vi "C867_Macro_Test.vi"() -> ()   [LabVIEW 2026]
panel:
  out "BOOL 5":i32
  out "BOOL 4":i32
  out "BOOL 3":i32
  out "BOOL 2":i32
  out "BOOL":i32
  out "szAnswer":string
  out "error out":errorcluster caption="sortie d'erreur"
  in  "error in":errorcluster caption="entrée d'erreur"
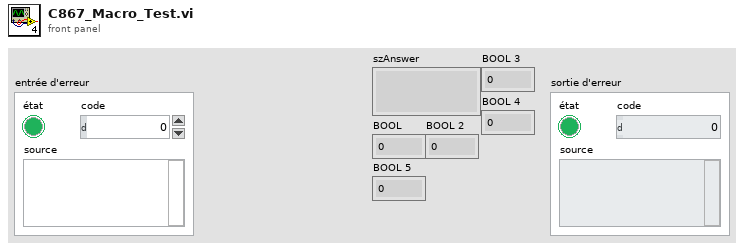
[diagram p1: front panel]
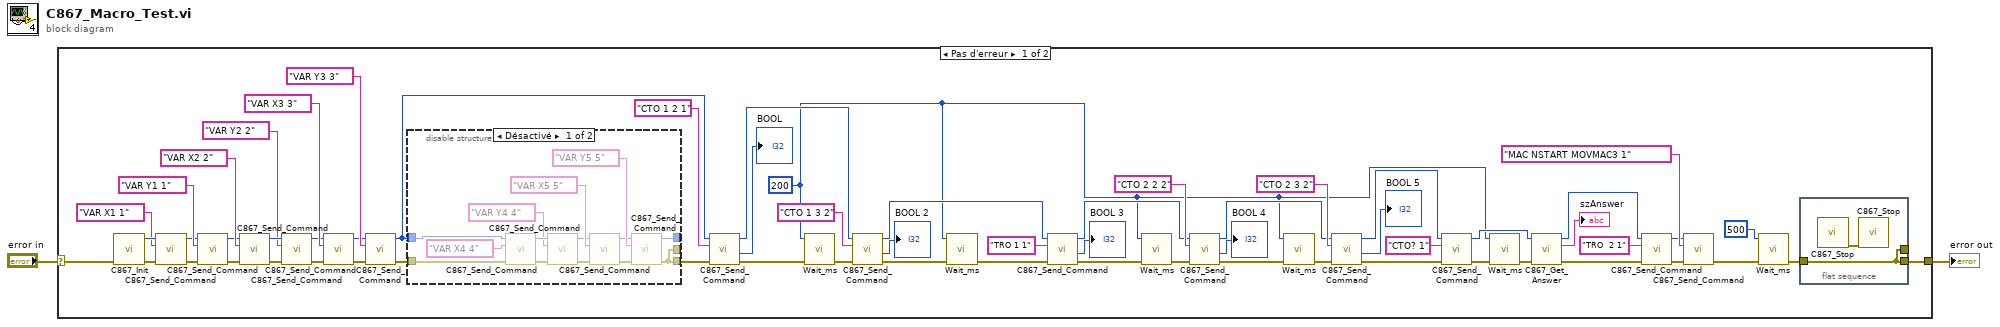
[diagram p0: block diagram]
diagram:
  n1 = case shown="Pas d'erreur" "error in" {
    selector: "error in" -> [w64 w83]
    tunnel: [w42 w83] -> w1
    frame No Error {
      w19 = u32 200 ("milliseconds to wait")
      n2 = call "C867_Init.vi"("error in"=w64) -> ("error out"=w62:errorcluster, "ID"=w61:i32)  [unwired: 9 in]
      n3 = call "C867_Send_Command.vi"("entrée d'erreur (pas d'erreur)"=w62, "szCommand"="VAR X1 1", "ID en entrée"=w61) -> ("sortie d'erreur"=w58:errorcluster, "ID en sortie"=w55:i32)  [unwired: 5 in, 2 out]
      n4 = call "C867_Send_Command.vi"("entrée d'erreur (pas d'erreur)"=w58, "szCommand"="VAR Y1 1", "ID en entrée"=w55) -> ("sortie d'erreur"=w46:errorcluster, "ID en sortie"=w45:i32)  [unwired: 5 in, 2 out]
      n5 = call "C867_Send_Command.vi"("entrée d'erreur (pas d'erreur)"=w46, "szCommand"="VAR X2 2", "ID en entrée"=w45) -> ("sortie d'erreur"=w53:errorcluster, "ID en sortie"=w54:i32)  [unwired: 5 in, 2 out]
      n6 = call "C867_Send_Command.vi"("entrée d'erreur (pas d'erreur)"=w53, "szCommand"="VAR Y2 2", "ID en entrée"=w54) -> ("sortie d'erreur"=w43:errorcluster, "ID en sortie"=w44:i32)  [unwired: 5 in, 2 out]
      n7 = call "C867_Send_Command.vi"("entrée d'erreur (pas d'erreur)"=w43, "szCommand"="VAR X3 3", "ID en entrée"=w44) -> ("sortie d'erreur"=w48:errorcluster, "ID en sortie"=w47:i32)  [unwired: 5 in, 2 out]
      n8 = call "C867_Send_Command.vi"("entrée d'erreur (pas d'erreur)"=w48, "szCommand"="VAR Y3 3", "ID en entrée"=w47) -> ("sortie d'erreur"=w41:errorcluster, "ID en sortie"=w5:i32)  [unwired: 5 in, 2 out]
      n9 = disable-structure shown="Désactivé" {
        disable-tunnel: w41 -> [w70 w80]
        disable-tunnel: [w65 w80] -> _
        disable-tunnel: [w68 w79] -> _
        disable-tunnel: w5 -> [w66 w79]
        disable-tunnel: [w65 _] -> w6
        frame Disabled {
          n10 = call "C867_Send_Command.vi"("entrée d'erreur (pas d'erreur)"=w70, "szCommand"="VAR X4 4", "ID en entrée"=w66) -> ("sortie d'erreur"=w77:errorcluster, "ID en sortie"=w78:i32)  [unwired: 5 in, 2 out]
          n11 = call "C867_Send_Command.vi"("entrée d'erreur (pas d'erreur)"=w77, "szCommand"="VAR Y4 4", "ID en entrée"=w78) -> ("sortie d'erreur"=w69:errorcluster, "ID en sortie"=w67:i32)  [unwired: 5 in, 2 out]
          n12 = call "C867_Send_Command.vi"("entrée d'erreur (pas d'erreur)"=w69, "szCommand"="VAR X5 5", "ID en entrée"=w67) -> ("sortie d'erreur"=w72:errorcluster, "ID en sortie"=w71:i32)  [unwired: 5 in, 2 out]
          n13 = call "C867_Send_Command.vi"("entrée d'erreur (pas d'erreur)"=w72, "szCommand"="VAR Y5 5", "ID en entrée"=w71) -> ("sortie d'erreur"=w65:errorcluster, "ID en sortie"=w68:i32)  [unwired: 5 in, 2 out]
        }
        frame Enabled {
        }
      }
      n14 = call "C867_Send_Command.vi"("entrée d'erreur (pas d'erreur)"=w6, "szCommand"="CTO 1 2 1", "ID en entrée"=w5) -> ("sortie d'erreur"=w20:errorcluster, "BOOL"=→"BOOL":i32, "ID en sortie"=w33:i32)  [unwired: 5 in, 1 out]
      n15 = call "Wait_ms.vi"("error in (no error)"=w20, "milliseconds to wait"=w19) -> ("error out"=w21:errorcluster)  [unwired: 9 in]
      n16 = call "C867_Send_Command.vi"("entrée d'erreur (pas d'erreur)"=w21, "szCommand"="CTO 1 3 2", "ID en entrée"=w33) -> ("sortie d'erreur"=w18:errorcluster, "BOOL"=→"BOOL 2":i32, "ID en sortie"=w32:i32)  [unwired: 5 in, 1 out]
      n17 = call "Wait_ms.vi"("error in (no error)"=w18, "milliseconds to wait"=w19) -> ("error out"=w17:errorcluster)  [unwired: 9 in]
      n18 = call "C867_Send_Command.vi"("entrée d'erreur (pas d'erreur)"=w17, "szCommand"="TRO 1 1", "ID en entrée"=w32) -> ("sortie d'erreur"=w16:errorcluster, "BOOL"=→"BOOL 3":i32, "ID en sortie"=w31:i32)  [unwired: 5 in, 1 out]
      n19 = call "Wait_ms.vi"("error in (no error)"=w16, "milliseconds to wait"=w19) -> ("error out"=w15:errorcluster)  [unwired: 9 in]
      n20 = call "C867_Send_Command.vi"("entrée d'erreur (pas d'erreur)"=w15, "szCommand"="CTO 2 2 2", "ID en entrée"=w31) -> ("sortie d'erreur"=w14:errorcluster, "BOOL"=→"BOOL 4":i32, "ID en sortie"=w30:i32)  [unwired: 5 in, 1 out]
      n21 = call "Wait_ms.vi"("error in (no error)"=w14, "milliseconds to wait"=w19) -> ("error out"=w13:errorcluster)  [unwired: 9 in]
      n22 = call "C867_Send_Command.vi"("entrée d'erreur (pas d'erreur)"=w13, "szCommand"="CTO 2 3 2", "ID en entrée"=w30) -> ("sortie d'erreur"=w12:errorcluster, "BOOL"=→"BOOL 5":i32, "ID en sortie"=w29:i32)  [unwired: 5 in, 1 out]
      n23 = call "C867_Send_Command.vi"("entrée d'erreur (pas d'erreur)"=w12, "szCommand"="CTO? 1", "ID en entrée"=w29) -> ("sortie d'erreur"=w22:errorcluster, "ID en sortie"=w27:i32)  [unwired: 5 in, 2 out]
      n24 = call "Wait_ms.vi"("error in (no error)"=w22, "milliseconds to wait"=w19) -> ("error out"=w23:errorcluster)  [unwired: 9 in]
      n25 = call "C867_Get_Answer.vi"("entrée d'erreur (pas d'erreur)"=w23, "ID en entrée"=w27) -> ("sortie d'erreur"=w25:errorcluster, "szAnswer"=→"szAnswer":string, "ID en sortie"=w26:i32)  [unwired: 6 in, 1 out]
      n26 = call "C867_Send_Command.vi"("entrée d'erreur (pas d'erreur)"=w25, "szCommand"="TRO  2 1", "ID en entrée"=w26) -> ("sortie d'erreur"=w4:errorcluster, "ID en sortie"=w3:i32)  [unwired: 5 in, 2 out]
      n27 = call "C867_Send_Command.vi"("entrée d'erreur (pas d'erreur)"=w4, "szCommand"="MAC NSTART MOVMAC3 1", "ID en entrée"=w3) -> ("sortie d'erreur"=w56:errorcluster)  [unwired: 5 in, 3 out]
      n28 = call "Wait_ms.vi"("error in (no error)"=w56, "milliseconds to wait"=u32 500) -> ("error out"=w40:errorcluster)  [unwired: 9 in]
      n29 = flat-sequence {
        tunnel: [w81] -> _
        tunnel: [w81] -> w42
        tunnel: w40 -> [w81]
        frame #0 {
          n30 = call "C867_Stop.vi"() -> ("error out"=w82:errorcluster)  [unwired: 11 in]
          n31 = call "C867_Stop.vi"("error in"=w82) -> ()  [unwired: 10 in, 1 out]
        }
      }
    }
    frame Error {
    }
  }
  "error out" <- w1
